vi "Event Handler Dispatcher.vi"(8 "error in (no error)":errorcluster, 11 "Control in":refnum<class "Control.lvclass">) -> (0 "error out":errorcluster)   [LabVIEW 2023, in "Control.lvclass"]
doc: "The Event Handler Dispatch then has three purposes:\n\nFirst, it creates a \"Stop\" User Event that must be registered for in every Event Handler.\n\nSecond, it asynchronously launches the Orphan Check.vi. The Orphan Check VI watches the Live Caller Queue. When the queue goes invalid, it generates the \"Stop\" User Event.\n\nThird, after the Orphan Check VI is launched and running, the Event Handler is called. Because Event Handler is dynamic dispatched it will call the one for the given class.\n\nThe Event Handler Dispatcher waits here until the Event Handler finishes by events in its code or the \"Stop\" User Event\n<b> </b> <b> </b>\n©2016 Q Software Innovations, LLC (QSI)\nwritten by Quentin Alldredge\nproduced in LabVIEW 2015\n\nsupport@qsoftwareinnovations.com\nwww.qsoftwareinnovations.com\n\nAll rights reserved.\n\nRedistribution and use in source and binary forms, with or without modification, are permitted provided that the following conditions are met:\n\n * Redistributions of source code must retain the above copyright notice, this list of conditions and the following disclaimer.\n * Redistributions in binary form must reproduce the above copyright notice, this list of conditions and the following disclaimer in the documentation and/or other materials provided with the distribution.\n * Neither the name of Q Software Innovations, LLC. nor the names of its contributors may be used to endorse or promote products derived from this software without specific prior written permission.\n\nTHIS SOFTWARE IS PROVIDED BY THE COPYRIGHT HOLDERS AND CONTRIBUTORS \"AS IS\" AND ANY EXPRESS OR IMPLIED WARRANTIES, INCLUDING, BUT NOT LIMITED TO, THE IMPLIED WARRANTIES OF MERCHANTABILITY AND FITNESS FOR A PARTICULAR PURPOSE ARE DISCLAIMED. IN NO EVENT SHALL THE COPYRIGHT OWNER OR CONTRIBUTORS BE LIABLE FOR ANY DIRECT, INDIRECT, INCIDENTAL, SPECIAL, EXEMPLARY, OR CONSEQUENTIAL DAMAGES (INCLUDING, BUT NOT LIMITED TO, PROCUREMENT OF SUBSTITUTE GOODS OR SERVICES; LOSS OF USE, DATA, OR PROFITS; OR BUSINESS INTERRUPTION) HOWEVER CAUSED AND ON ANY THEORY OF LIABILITY, WHETHER IN CONTRACT, STRICT LIABILITY, OR TORT (INCLUDING NEGLIGENCE OR OTHERWISE) ARISING IN ANY WAY OUT OF THE USE OF THIS SOFTWARE, EVEN IF ADVISED OF THE POSSIBILITY OF SUCH DAMAGE."
uses:
  Control.lvclass
  Control.lvclass/Control.ctl
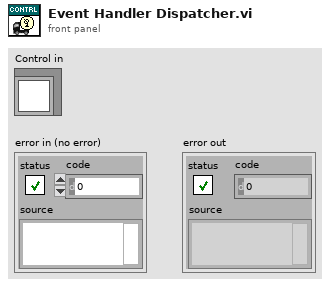
[diagram p1: front panel]
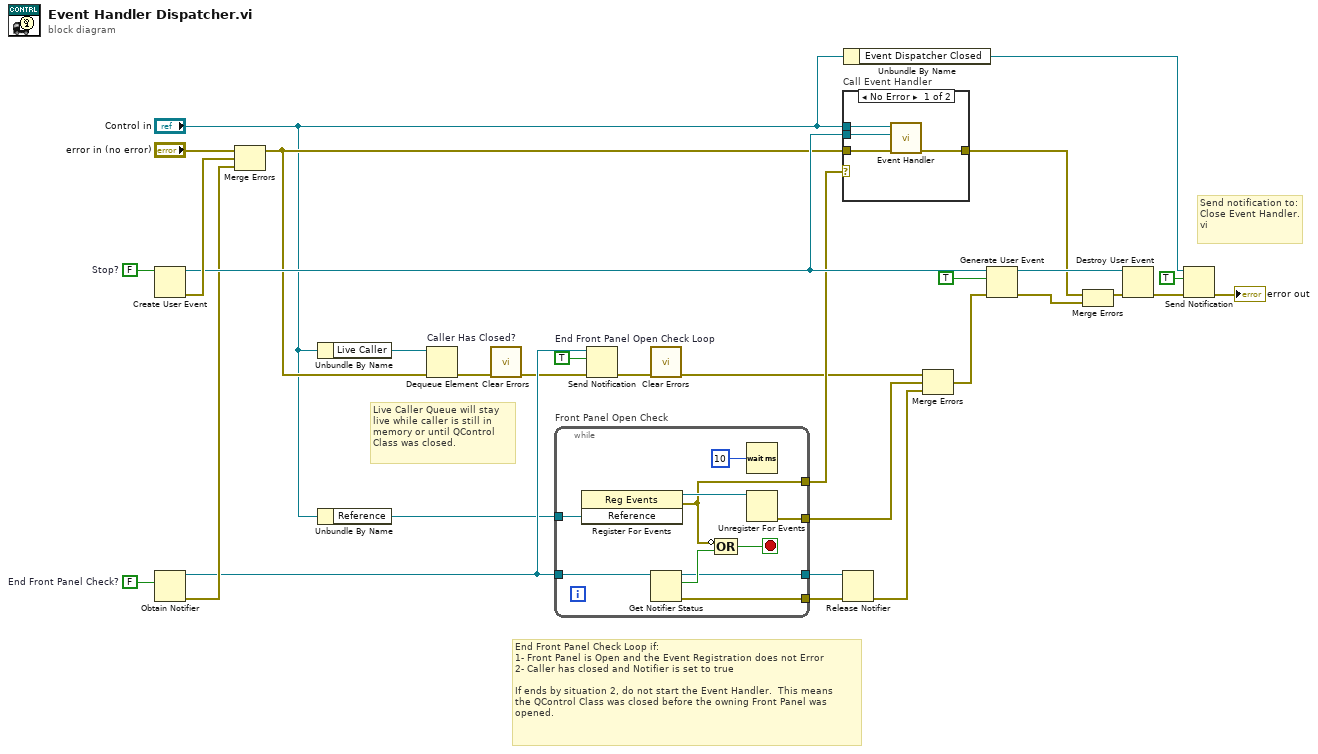
[diagram p0: block diagram]
diagram:
  w21 = FALSE  # End Front Panel Check?
  w30 = FALSE  # Stop?
  # "Send notification to: Close Event Handler.vi"
  # "Live Caller Queue will stay \nlive while caller is still in \nmemory or until QControl \nClass was closed."
  # "End Front Panel Check Loop if:\n1- Front Panel is Open and the Event Registration does not Error\n2- Caller has closed and Notifier is set to true\n\nIf ends by situation 2, do not start the Event Handler.  This means\nthe QControl Class was closed before the owning Front Panel was\nopened."
  n1 = Create User Event(user event datatype=w30) -> (user event=w24:refnum<user-event>, error out=w29:errorcluster)  [unwired: 1 in]
  n2 = Obtain Notifier(notification data type=w21) -> (notifier out=w19:refnum<notifier>, error out=w20:errorcluster)  [unwired: 3 in, 1 out]
  n3 = Merge Errors("error in (no error)", w29, w20) -> (w7:errorcluster)
  n4 = Unbundle By Name("Control in") -> ("Live Caller"=w12:refnum<queue>)
  n5 = Unbundle By Name("Control in") -> ("Reference"=w11:refnum<vi>)
  n6 = Dequeue Element "Caller Has Closed?"(queue=w12, error in (no error)=w7) -> (error out=w27:errorcluster)  [unwired: 1 in, 3 out]
  n7 = call <vilib>:"Clear Errors.vi"("error in (no error)"=w27) -> ("error out"=w14:errorcluster)  [unwired: 5 in, 1 out]
  n8 = while "Front Panel Open Check" {
    tunnel: w11 -> [w41]
    tunnel: [w33] -> w22
    tunnel: w19 -> [w39]
    tunnel: [w37] -> w16
    tunnel: [w35] -> w10
    tunnel: [w32] -> w8
    stop <- w40 stop-if-true
    n9 = register-events(w41) -> (reference out=w34:refnum<event-registration>, error out=w33:errorcluster)  [unwired: 2 in]
    n10 = Get Notifier Status(notifier=w39) -> (notifier out=w37:refnum<notifier>, current notification=w38:bool, error out=w35:errorcluster)  [unwired: 1 in, 2 out]
    n11 = Compound Arithmetic op=OR(invert w33, w38) -> (w40:bool)
    n12 = Wait (ms)(milliseconds to wait=u32 10) -> ()  [unwired: 1 out]
    n13 = Unregister For Events(event registration refnum=w34) -> (error out=w32:errorcluster)  [unwired: 1 in]
  }
  n14 = Send Notification "End Front Panel Open Check Loop"(notification=TRUE, notifier=w19, error in (no error)=w14) -> (error out=w17:errorcluster)  [unwired: 1 out]
  n15 = call <vilib>:"Clear Errors.vi"("error in (no error)"=w17) -> ("error out"=w13:errorcluster)  [unwired: 5 in, 1 out]
  n16 = case "Call Event Handler" shown="No Error" w22 {
    tunnel: [w45 w46] -> w6
    tunnel: w7 -> [w44 w46]
    tunnel: "Control in" -> [w43 _]
    tunnel: w24 -> [w42 _]
    frame No Error {
      n17 = call-dynamic "Event Handler.vi"("error in (no error)"=w44, "Stop Event Hander"=w42, "Control in"=w43) -> ("error out"=w45:errorcluster)  [unwired: 8 in]
    }
    frame Error {
    }
  }
  n18 = Release Notifier(notifier=w16, error in (no error)=w10) -> (error out=w15:errorcluster)  [unwired: 1 in, 2 out]
  n19 = Unbundle By Name("Control in") -> ("Event Dispatcher Closed"=w3:refnum<notifier>)
  n20 = Merge Errors(w13, w8, w15) -> (w9:errorcluster)
  n21 = Generate User Event(user event=w24, event data cluster=TRUE ("event data"), error in=w9) -> (user event out=w23:refnum<user-event>, error out=w25:errorcluster)  [unwired: 1 in]
  n22 = Merge Errors(w6, w25) -> (w28:errorcluster)
  n23 = Destroy User Event(user event=w23, error in=w28) -> (error out=w5:errorcluster)
  n24 = Send Notification(notification=TRUE, notifier=w3, error in (no error)=w5) -> (error out=→"error out":errorcluster)  [unwired: 1 out]
